vi "GA Get Lmt Sns.vi"(8 "error in (no error)":errorcluster caption="错误输入（无错误）", 11 "pSense":u16) -> (0 "error out":errorcluster caption="错误输出", 2 "function return":i32, 3 "pSense out":u16)   [LabVIEW 2015, in "GAS.lvlib"]
doc: "extern \"C\" __declspec(dllimport) int GA_GetLmtSns(unsigned short *pSense);"
uses:
  <userlib>/BP_GAS/GAS.lvlib
  <userlib>/BP_GAS/GAS.dll
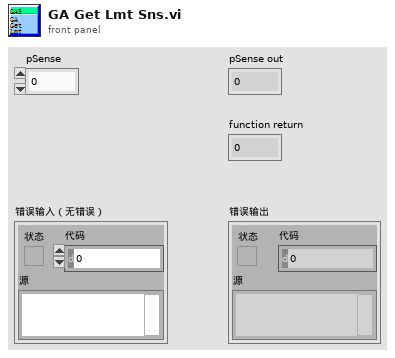
[diagram p1: front panel]
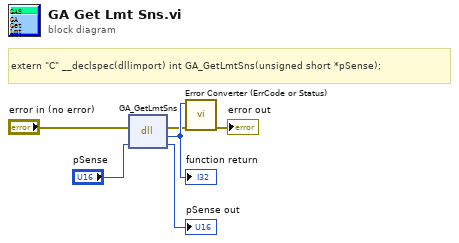
[diagram p0: block diagram]
diagram:
  # "extern \"C\" __declspec(dllimport) int GA_GetLmtSns(unsigned short *pSense);"
  n1 = dll-call lib="E:/Program Files (x86)/National Instruments/LabVIEW 2015/user.lib/BP_GAS/GAS.*" fn="GA_GetLmtSns"(error in="error in (no error)", "pSense"="pSense") -> (error out=w2:errorcluster, w6:i32, "pSense"=→"pSense out":u16)  [unwired: 2 in, 1 out]
  "function return" <- w6
  n2 = call "Error Converter (ErrCode or Status).vi"("error in (no error)"=w2, "error code"=w6) -> ("error out"=→"error out":errorcluster)  [unwired: 9 in]
